vi "AppendNode.vi"(8 "Error In":errorcluster, 10 "Child Node":refnum<k20>, 11 "Parent Node In":refnum<k20>) -> (0 "Error Out":errorcluster, 3 "Parent Node Out":refnum<k20>)   [LabVIEW 2012, in "LV-Utilities.lvlib"]
uses:
  LV-Utilities.lvlib
  <resource>/objmgr/DOMUserDefRef.rc
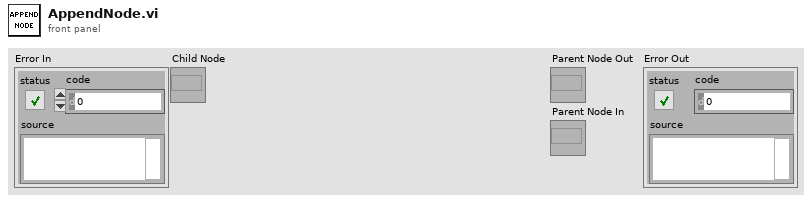
[diagram p1: front panel]
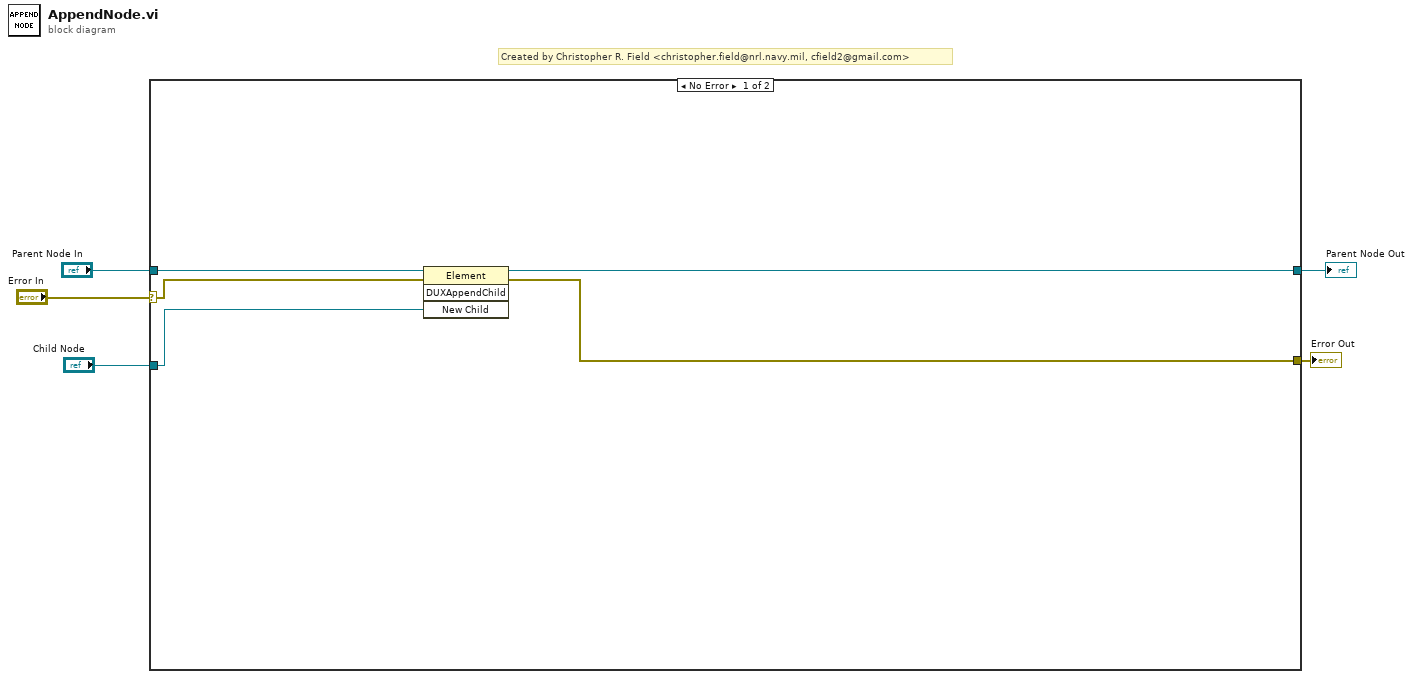
[diagram p0: block diagram]
diagram:
  # "Created by Christopher R. Field <christopher.field@nrl.navy.mil, cfield2@gmail.com>"
  n1 = case shown="No Error" "Error In" {
    selector: "Error In" -> [w8 w11]
    tunnel: "Parent Node In" -> [w10 w12]
    tunnel: [w9 w12] -> w4
    tunnel: "Child Node" -> [w7 _]
    tunnel: [w6 w11] -> w1
    frame No Error {
      n2 = invoke class="Element" method="DUXAppendChild"(reference=w10, error in=w8, "New Child"=w7) -> (reference out=w9:refnum<k20>, error out=w6:errorcluster)  [unwired: 1 in, 2 out]
    }
    frame Error {
    }
  }
  "Parent Node Out" <- w4
  "Error Out" <- w1
